vi "Chroma 1905x Series Memory Free State query.vi"(7 "error in (no error)":errorcluster, 10 "VISA resource name":refnum<visa-resource-name>) -> (0 "error out":errorcluster, 3 "VISA resource name out":refnum<visa-resource-name>, 9 "Result":string)   [LabVIEW 2025]
doc: "Contact Chroma\nTEL: +886-2-2298-3855 \nTEL: +886-3-397-5788 \nFAX: +886-2-2298-3596\nFAX: +886-3-327-4703 \nURL: http://www.chromaate.com \nE-mail: chroma@chroma.com.tw"
uses:
  <instrlib>/Chroma 19052/Chroma 19052.lvlib
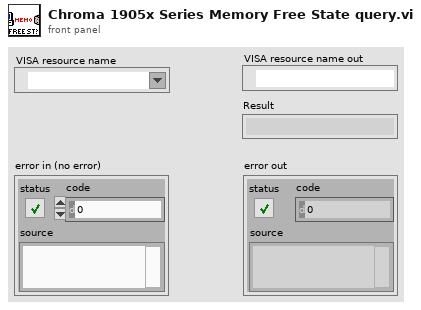
[diagram p1: front panel]
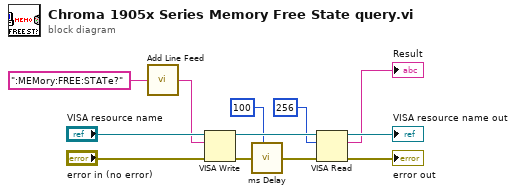
[diagram p0: block diagram]
diagram:
  n1 = call <instrlib>:"Add Line Feed.vi"("Command string"=":MEMory:FREE:STATe?") -> ("Concatenated string"=w7:string)  [unwired: 4 in]
  n2 = VISA Write(VISA resource name="VISA resource name", write buffer=w7, error in (no error)="error in (no error)") -> (VISA resource name out=w12:refnum<visa-resource-name>, error out=w5:errorcluster)  [unwired: 1 out]
  n3 = call <instrlib>:"ms Delay.vi"("miliseconds to wait"=u32 100 ("Time Delay ms"), "error in (no error)"=w5) -> ("error out"=w6:errorcluster)  [unwired: 6 in, 1 out]
  n4 = VISA Read(VISA resource name=w12, byte count=u32 256, error in (no error)=w6) -> (VISA resource name out=→"VISA resource name out":refnum<visa-resource-name>, read buffer=→"Result":string, error out=→"error out":errorcluster)  [unwired: 1 out]
